vi "save_state.vi"(0 "state":u16(ring) items=["none", "walking", "bicycling", "stairs up"], 2 "peaks":dbl[][](array[numeric])) -> ()   [LabVIEW 2009]
uses:
  activity_info.vi
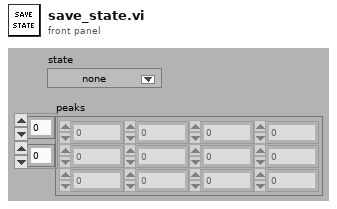
[diagram p1: front panel]
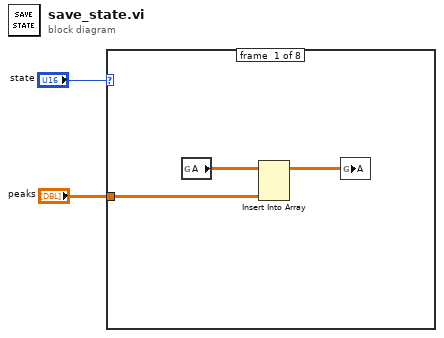
[diagram p0: block diagram]
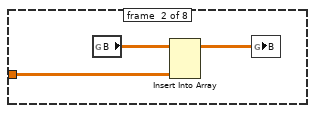
[diagram p2: hidden frame]
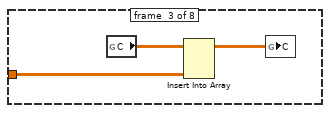
[diagram p3: hidden frame]
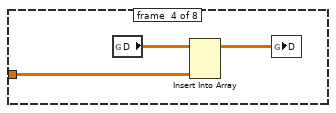
[diagram p4: hidden frame]
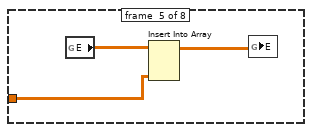
[diagram p5: hidden frame]
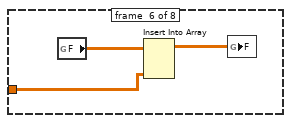
[diagram p6: hidden frame]
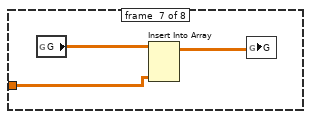
[diagram p7: hidden frame]
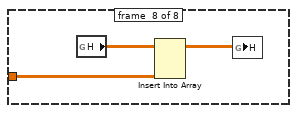
[diagram p8: hidden frame]
diagram:
  n1 = case shown="7" "state" {
    tunnel: "peaks" -> [w5 w6 w9 w12 w16 w18 w22 w26]
    frame #0 {
      n2 = global read "activity_info.vi" "A"() -> (w4:dbl[][])
      n3 = Insert Into Array(array=w4, new element=w5) -> (w3:dbl[][])  [unwired: 2 in]
      n4 = global write "activity_info.vi" "A"(w3) -> ()
    }
    frame #1 {
      n5 = global read "activity_info.vi" "B"() -> (w8:dbl[][])
      n6 = Insert Into Array(array=w8, new element=w6) -> (w7:dbl[][])  [unwired: 2 in]
      n7 = global write "activity_info.vi" "B"(w7) -> ()
    }
    frame #2 {
      n8 = global read "activity_info.vi" "C"() -> (w11:dbl[][])
      n9 = Insert Into Array(array=w11, new element=w9) -> (w10:dbl[][])  [unwired: 2 in]
      n10 = global write "activity_info.vi" "C"(w10) -> ()
    }
    frame #3 {
      n11 = global read "activity_info.vi" "D"() -> (w14:dbl[][])
      n12 = Insert Into Array(array=w14, new element=w12) -> (w13:dbl[][])  [unwired: 2 in]
      n13 = global write "activity_info.vi" "D"(w13) -> ()
    }
    frame #4 {
      n14 = global read "activity_info.vi" "E"() -> (w17:dbl[][])
      n15 = Insert Into Array(array=w17, new element=w16) -> (w15:dbl[][])  [unwired: 2 in]
      n16 = global write "activity_info.vi" "E"(w15) -> ()
    }
    frame #5 {
      n17 = global read "activity_info.vi" "F"() -> (w20:dbl[][])
      n18 = Insert Into Array(array=w20, new element=w18) -> (w19:dbl[][])  [unwired: 2 in]
      n19 = global write "activity_info.vi" "F"(w19) -> ()
    }
    frame #6 {
      n20 = global read "activity_info.vi" "G"() -> (w23:dbl[][])
      n21 = Insert Into Array(array=w23, new element=w22) -> (w21:dbl[][])  [unwired: 2 in]
      n22 = global write "activity_info.vi" "G"(w21) -> ()
    }
    frame #7 {
      n23 = global read "activity_info.vi" "H"() -> (w25:dbl[][])
      n24 = Insert Into Array(array=w25, new element=w26) -> (w24:dbl[][])  [unwired: 2 in]
      n25 = global write "activity_info.vi" "H"(w24) -> ()
    }
  }
